vi "Stop Test.vi"(8 "error in (no error)":errorcluster, 11 "Execution Profiler In":refnum<class "Execution Profiler.lvclass">) -> (0 "error out":errorcluster, 3 "Execution Profiler Out":refnum<class "Execution Profiler.lvclass">)   [LabVIEW 2020, in "Execution Profiler.lvlib" / "Execution Profiler.lvclass"]
uses:
  Execution Profiler.lvclass
  Execution Profiler.lvclass/Execution Profiler.ctl
  Execution Profiler View.vi
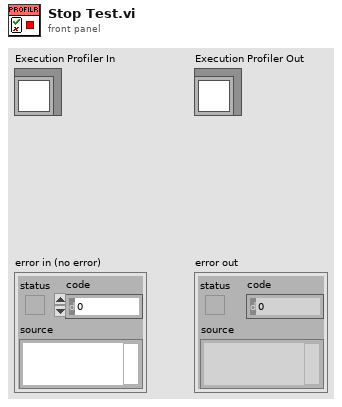
[diagram p1: front panel]
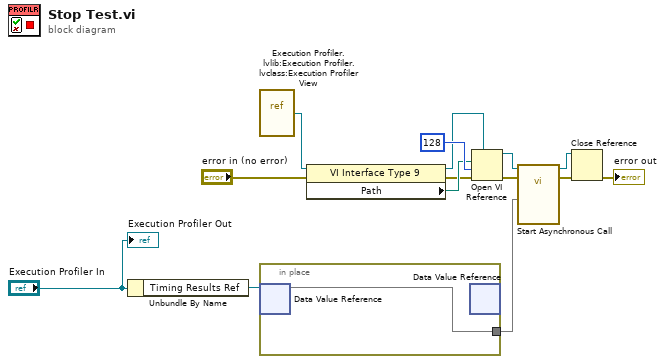
[diagram p0: block diagram]
diagram:
  n1 = Unbundle By Name("Execution Profiler In") -> ("Timing Results Ref"=w1:refnum<data-value>)
  n2 = vi-ref "Execution Profiler.lvlib:Execution Profiler.lvclass:Execution Profiler View.vi"() -> (w9:refnum<vi>)
  n3 = in-place {
    in-place-border: [w15] -> w2
    n4 = in-place-dvr #1(w1) -> (w15:map{string, dbl})  [unwired: 1 out]
    n5 = in-place-dvr #1() -> ()  [unwired: 1 in, 2 out]
  }
  n6 = property class="VI Interface Type 9"(reference=w9, error in="error in (no error)") -> (reference out=w11:refnum<vi>, error out=w7:errorcluster, "Path"=w10:path)
  n7 = Open VI Reference(type specifier VI Refnum (for type only)=w11, vi path=w10, options=128, error in (no error)=w7) -> (vi reference=w8:refnum<vi>, error out=w3:errorcluster)  [unwired: 2 in]
  n8 = call-by-ref "Start Asynchronous Call"(reference=w8, error in=w3, "Timing Results"=w2) -> (reference out=w14:refnum<vi>, error out=w13:errorcluster)  [unwired: 10 in, 1 out]
  n9 = Close Reference(reference=w14, error in (no error)=w13) -> (error out=→"error out":errorcluster)
  "Execution Profiler Out" <- "Execution Profiler In"
